vi "Create.vi"(5 "REST Client Headers_NET in":refnum<class "REST Client Headers_NET.lvclass">, 8 "error in (no error)":errorcluster, 11 "Headers":T1) -> (0 "error out":errorcluster, 3 "REST Client Headers_NET out":refnum<class "REST Client Headers_NET.lvclass">)   [LabVIEW 2018, in "REST Client_NET.lvlib" / "REST Client Headers_NET.lvclass"]
doc: "<b> </b> <b> </b>\nHttpClient_NET\nJustin Young - Viviota\nCopyright (c) 2021\nLicense: BSD"
uses:
  REST Client Headers_NET.lvclass
  Types/ResponseHeaders_Cluster.ctl
  HttpHeaders_response/HttpHeaders_Response.lvclass
  HttpHeaders_content/HttpHeaders_Content.lvclass
  REST Client Headers_NET.lvclass/REST Client Headers_NET.ctl
  HttpClient_NET.lvlib
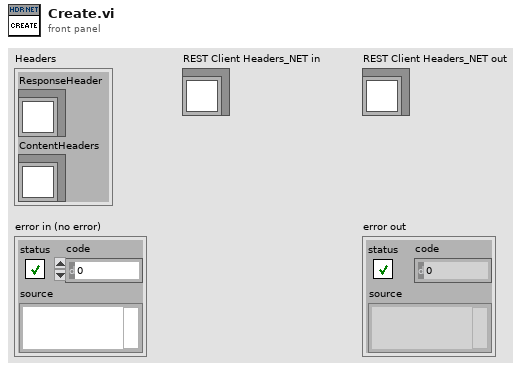
[diagram p1: front panel]
types:
  T1 = typedef "HttpClient_NET.lvlib/ResponseHeaders_Cluster.ctl" = cluster{"ResponseHeader":refnum<class "HttpHeaders_Response.lvclass">, "ContentHeaders":refnum<class "HttpHeaders_Content.lvclass">}
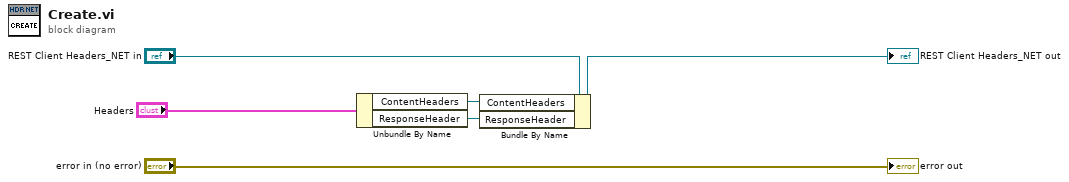
[diagram p0: block diagram]
diagram:
  n1 = Unbundle By Name("Headers") -> ("ContentHeaders"=w2:refnum<class "HttpHeaders_Content.lvclass">, "ResponseHeader"=w1:refnum<class "HttpHeaders_Response.lvclass">)
  n2 = Bundle By Name(cluster="REST Client Headers_NET in", "ContentHeaders"=w2, "ResponseHeader"=w1) -> (→"REST Client Headers_NET out":refnum<class "REST Client Headers_NET.lvclass">)
  "error out" <- "error in (no error)"
